vi "Robotics Environment Simulator.vi"() -> ()   [LabVIEW 2013]
doc: "This VI starts and stops the environment simulator and serves as the master VI for your simulation code. Open and run this VI to display the environment simulator, or open the block diagram to view or modify simulation code."
uses:
  <vilib>/Analysis/Matrix/Datatypes/RealMatrix.ctl
  <vilib>/robotics/Simulator/Engine/ctl/Step Mode.ctl
  <vilib>/robotics/Simulator/Engine/ctl/Simulation Mode.ctl
  <vilib>/robotics/Simulator/Engine/ctl/Robot Component ID.ctl
  <resource>/robotics/simulator/Utility/ModelBuilder/Utilities/3DController/Public/ActionType.ctl
  <resource>/robotics/simulator/Utility/ModelBuilder/Utilities/3DController/3DController.lvclass
  SubVIs/SR6-NC Arm/SR6-NC Arm.lvclass
  <instrlib>/Hitec HS400 Series/HAIOL/Hitec HS400 Series.lvclass
  <vilib>/Analysis/baseanly.llb/Real A x B.vi
  <vilib>/Analysis/_algsub.llb/Vector Norm.vi
  <vilib>/Analysis/_algsub.llb/Real Vector Norm.vi
  <vilib>/Analysis/baseanly.llb/Outer Product.vi
  <vilib>/Analysis/baseanly.llb/Real Outer Product.vi
  <vilib>/robotics/Kinematics/Create Lie Group Matrix.vi
  <vilib>/robotics/Simulator/Interface/Simulator References/Get Robot Component Reference.vi
  <vilib>/robotics/Simulator/Interface/Simulator References/Get 3D Visual Scene Reference.vi
  <vilib>/Analysis/baseanly.llb/Real Inverse Matrix.vi
  <vilib>/Analysis/7linalg.llb/Create Special Matrix.vi
  <vilib>/Analysis/7linalg.llb/Create Special Real Matrix.vi
  <vilib>/Analysis/Matrix/Numeric/Multiply/Multiply.vi
  <vilib>/Analysis/Matrix/Numeric/Multiply/Multiply - RM,R.vi
  <vilib>/Analysis/Matrix/Numeric/Multiply/Multiply - R,RM.vi
  <vilib>/Analysis/Matrix/Numeric/Add/Add.vi
  <vilib>/Analysis/Matrix/Numeric/Add/Add - RM,RM.vi
  <vilib>/Analysis/Matrix/Numeric/Subtract/Subtract - RM,RM.vi
  <vilib>/robotics/Kinematics/Robot/Forward Kinematics (Point).vi
  <vilib>/robotics/Simulator/NI_Robotics_Simulator.lvlib
  <instrlib>/Hitec HS400 Series/HAIOL/Simulator/Hitec HS400 Series Simulator.lvclass
  <resource>/objmgr/LVODE.rc
  <vilib>/robotics/Kinematics/NI_Kinematics.lvlib
  <vilib>/Analysis/NI_AALBase.lvlib
  <vilib>/Analysis/Matrix/NI_Matrix.lvlib
panel:
  out "A - B 2":T1
  out "transform":T1
  out "A - B":T1
  out "end effector transform":T1
  out "Ttar":T1
  out "exit":bool
  out "3D Picture":refnum<vi>(3d-picture)
  in  "Joints":dbl[](array[slide])=[0.0, 0.0, 0.0, 0.0, 0.0, -3.673469387755098] scale=-180.0..180.0
  in  "manifest filename":string="Robotics Environment Simulator.xml"
  in  "stop":bool
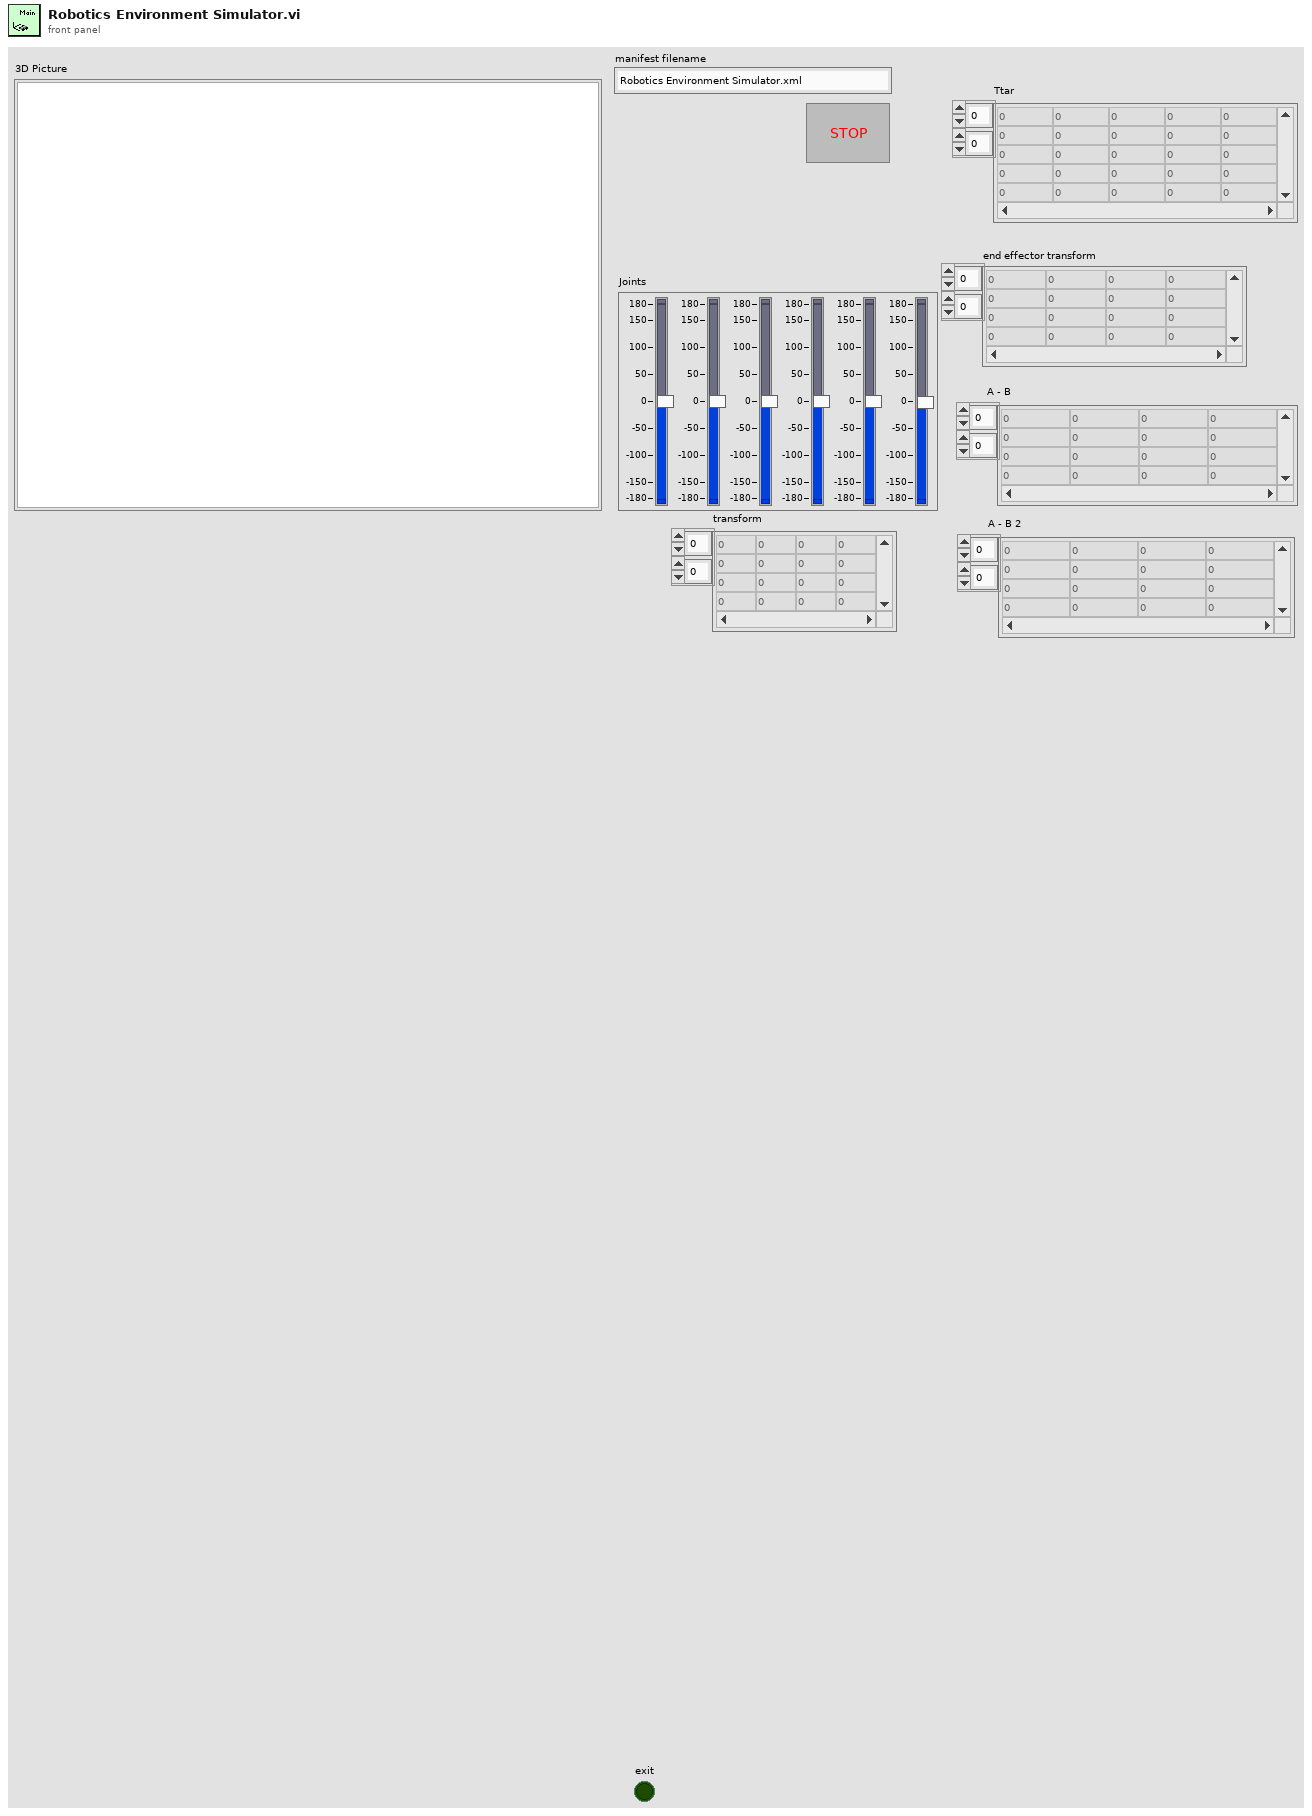
[diagram p1: front panel]
types:
  T1 = typedef "NI_Matrix.lvlib/RealMatrix.ctl" = dbl[][]
  T2 = typedef "NI_Robotics_Simulator.lvlib/Simulation Mode.ctl" = u16
  T3 = typedef "NI_Robotics_Simulator.lvlib/Step Mode.ctl" = u16
  T4 = typedef "NI_Robotics_Simulator.lvlib/Robot Component ID.ctl" = cluster{"robot ID":string, "component ID":string}
  T5 = typedef "NI_Robotics_Model_Builder.lvlib/3DController.lvclass/ActionType.ctl" = enum16{"None", "Trans_X", "Trans_Y", "Trans_Z", "Rot_X", "Rot_Y", "Rot_Z"}
  T6 = cluster{"vector[0]":dbl, "vector[1]":dbl, "vector[2]":dbl}
  T7 = cluster{"Position[0]":sgl, "Position[1]":sgl, "Position[2]":sgl}
  T8 = cluster{"vector":cluster{"vector[0]":dbl, "vector[1]":dbl, "vector[2]":dbl}, "angle":dbl}
  T9 = typedef "LVPoint32TypeDef.ctl" = cluster{"Horizontal":i32, "Vertical":i32}
  T10 = typedef "LV3DPointTypeDef.ctl" = cluster{"X":sgl, "Y":sgl, "Z":sgl}
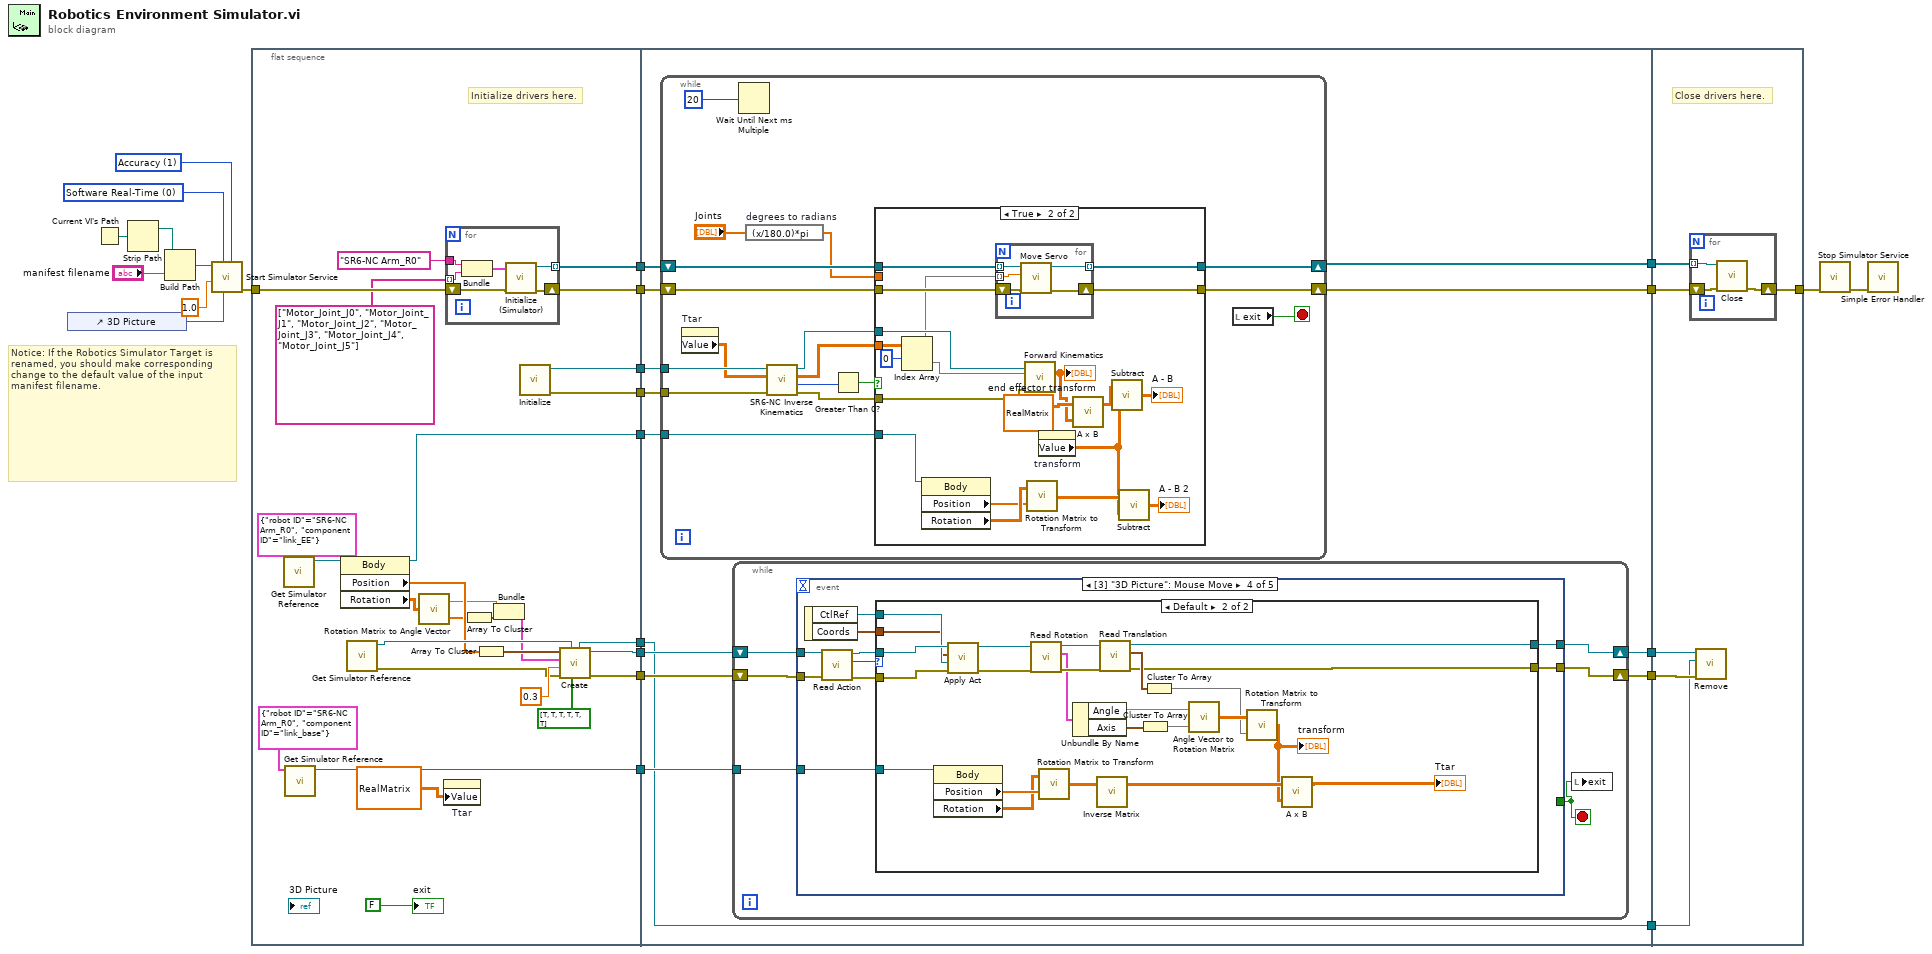
[diagram p0: block diagram]
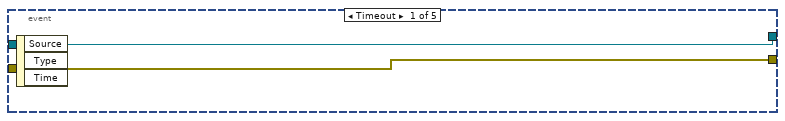
[diagram p2: hidden frame]
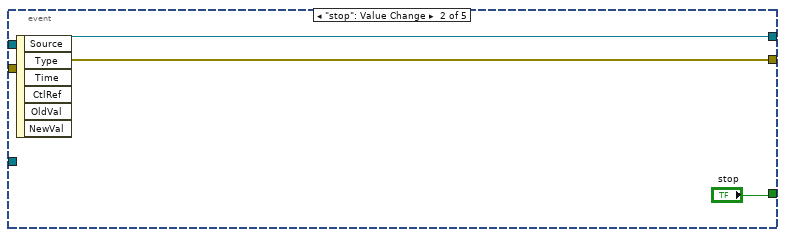
[diagram p3: hidden frame]
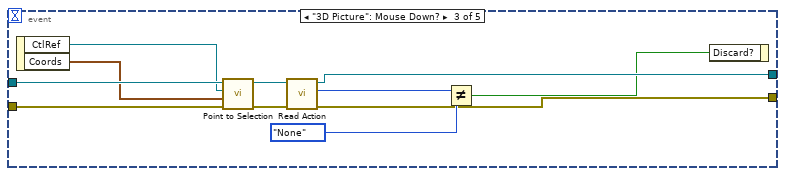
[diagram p4: hidden frame]
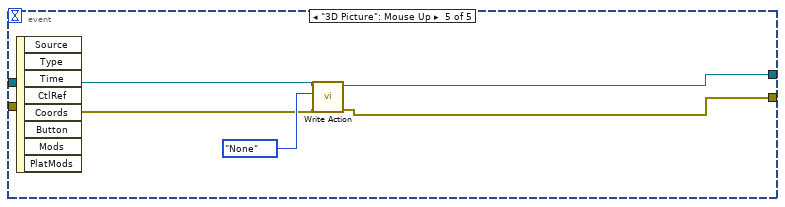
[diagram p6: hidden frame]
diagram:
  w12 = T2 0 items=["Software Real-Time", "Free Running", "Synchronized"] ("timing mode")
  w13 = T3 1 items=["Performance", "Accuracy"] ("step mode")
  # "Notice: If the Robotics Simulator Target is renamed, you should make corresponding change to the default value of the input manifest filename."
  n1 = control-ref of="3D Picture"() -> (w4:refnum<vi>)
  n2 = Current VI's Path() -> (path=w23:path)
  n3 = Strip Path(path=w23) -> (stripped path=w22:path)  [unwired: 1 out]
  n4 = Build Path(base path=w22, name or relative path="manifest filename") -> (appended path=w21:path)
  n5 = call <vilib>:"Start Simulator Service.vi"("step mode"=w13, "3D picture refnum"=w4, "timing mode"=w12, "step size (ms)"=1.0 ("stepsize(ms)"), "manifest file"=w21) -> ("error out"=w18:errorcluster)  [unwired: 6 in]
  n6 = flat-sequence {
    tunnel: w18 -> [w53]
    tunnel: [w52] -> w17
    tunnel: [w49] -> w15
    tunnel: [w35] -> w11
    tunnel: [w34] -> w10
    tunnel: [w33] -> w9
    tunnel: [w31] -> w8
    tunnel: [w29] -> w3
    tunnel: [w28] -> w2
    tunnel: [w26] -> w1
    tunnel: w17 -> [w71]
    tunnel: [w72] -> w16
    tunnel: w15 -> [w70]
    tunnel: [w69] -> w14
    tunnel: w11 -> [w63]
    tunnel: w10 -> [w67]
    tunnel: w9 -> [w68]
    tunnel: w8 -> [w66]
    tunnel: [w65] -> w7
    tunnel: [w64] -> w6
    tunnel: [w63] -> w5
    tunnel: w3 -> [w62]
    tunnel: w2 -> [w61]
    tunnel: w1 -> [w60]
    tunnel: [w182] -> w24
    tunnel: w16 -> [w183]
    tunnel: w14 -> [w184]
    tunnel: w7 -> [w181]
    tunnel: w6 -> [w180]
    tunnel: w5 -> [w179]
    frame #0 {
      # "Initialize drivers here."
      n7 = call-poly <vilib>:"Get Simulator Reference.vi"("robot component ID"=T4 {"robot ID"="SR6-NC Arm_R0", "component ID"="link_EE"}) -> ("component ref"=w42:refnum<k20>)  [unwired: 9 in, 1 out]
      n8 = call-poly <vilib>:"Get Simulator Reference.vi"("robot component ID"=T4 {"robot ID"="SR6-NC Arm_R0", "component ID"="link_base"}) -> ("component ref"=w31:refnum<k20>)  [unwired: 9 in, 1 out]
      n9 = property class="Body"(reference=w42) -> (reference out=w26:refnum<k20>, "Position"=w41:sgl[], "Rotation"=w40:sgl[][])  [unwired: 1 in, 1 out]
      n10 = call-poly <vilib>:"Get Simulator Reference.vi"() -> ("error out"=w43:errorcluster, "scene ref"=w44:refnum<vi>)  [unwired: 10 in]
      n11 = call <vilib>:"Rotation Matrix to Angle Vector.vi"("rotation matrix"=w40) -> ("angle"=w37:dbl, "vector"=w39:dbl[])
      n12 = property on="Ttar" class="Arr (strict)"("Value"=T1 [[1.0, 0.0, 0.0, 0.875], [0.0, 1.0, 0.0, 0.0], [0.0, 0.0, 1.0, 1.215], [0.0, 0.0, 0.0, 0.9999999999999997]] ("Ttar")) -> ()  [unwired: 2 in, 2 out]
      n13 = for {
        shift-right: [w58] -> w52
        shift-left: w53 -> [w59]
        tunnel: "SR6-NC Arm_R0" -> [w57]
        tunnel: string[] ["Motor_Joint_J0", "Motor_Joint_J1", "Motor_Joint_J2", "Motor_Joint_J3", "Motor_Joint_J4", "Motor_Joint_J5"] -> [w56] mode=indexing
        tunnel: [w54] -> w49 mode=indexing
        n14 = Bundle(w57, w56) -> (w55:cluster{string, string})  [unwired: 1 in]
        n15 = call <instrlib>:"Initialize (Simulator).vi"("error in (no error)"=w59, "Device ID"=w55) -> ("error out"=w58:errorcluster, "Hitec HS400 Series out"=w54:refnum<class "Hitec HS400 Series.lvclass">)  [unwired: 8 in]
      }
      n16 = Array To Cluster(array=w39) -> (cluster=w38:T6)
      n17 = Array To Cluster(array=w41) -> (cluster=w46:T7)
      n18 = Bundle("vector"=w38, "angle"=w37) -> (w36:T8)  [unwired: 1 in]
      n19 = call "Initialize.vi"() -> ("error out"=w28:errorcluster, "SR6-NC Arm out"=w29:refnum<class "SR6-NC Arm.lvclass">)  [unwired: 10 in]
      n20 = call <resource>:"Create.vi"("Marks"=bool[] [TRUE, TRUE, TRUE, TRUE, TRUE, TRUE], "Model Root"=w44, "error in (no error)"=w43, "Scale"=0.3, "Rotation"=w36, "Translation"=w46) -> ("error out"=w34:errorcluster, "3DController"=w33:refnum<class "3DController.lvclass">, "Model Root out"=w35:refnum<vi>)  [unwired: 3 in]
      "exit" <- FALSE ("exit")
    }
    frame #1 {
      n21 = while {
        shift-right: [w151] -> w72
        shift-left: w71 -> [w152]
        shift-right: [w149] -> w69
        shift-left: w70 -> [w150]
        tunnel: w62 -> [w144]
        tunnel: w61 -> [w143]
        tunnel: w60 -> [w136]
        stop <- w145 stop-if-true
        n22 = property on="Ttar" class="Arr (strict)"() -> ("Value"=w137:T1)  [unwired: 2 in, 2 out]
        n23 = Wait Until Next ms Multiple(millisecond multiple=20) -> ()  [unwired: 1 out]
        n24 = expression code="(x/180.0)*pi" "degrees to radians"("Joints") -> (w147:dbl[])
        n25 = call-dynamic "SR6-NC Inverse Kinematics.vi"("error in (no error)"=w143, "end effector transform"=w137, "SR6-NC Arm in"=w144) -> ("error out"=w138:errorcluster, "number of valid solutions"=w142:i32, "joint positions"=w140:T1, "SR6-NC Arm out"=w139:refnum<class "SR6-NC Arm.lvclass">)  [unwired: 5 in]
        n26 = Greater Than 0?(x=w142) -> (x > 0?=w141:bool)
        n27 = case shown="True" w141 {
          tunnel: w152 -> [w153 w173]
          tunnel: [w153 w172] -> w151
          tunnel: w150 -> [w154 w171]
          tunnel: [w154 w170] -> w149
          tunnel: w147 -> [_ _]
          tunnel: w140 -> [_ w169]
          tunnel: w139 -> [_ w167]
          tunnel: w138 -> [_ w165]
          tunnel: w136 -> [_ w158]
          frame False {
          }
          frame True {
            n28 = Index Array(array=w169, index (row)=0) -> (element=w166:dbl[])  [unwired: 1 in]
            n29 = property class="Body"(reference=w158) -> ("Position"=w159:sgl[], "Rotation"=w160:sgl[][])  [unwired: 1 in, 2 out]
            n30 = for {
              tunnel: w171 -> [w177] mode=indexing
              shift-right: [w176] -> w172
              shift-left: w173 -> [w178]
              tunnel: [w175] -> w170 mode=indexing
              tunnel: w166 -> [w174] mode=indexing
              n31 = call-dynamic "Move Servo.vi"("error in (no error)"=w178, "CCW Position (0.0 rad)"=w174, "Hitec HS400 Series in"=w177) -> ("error out"=w176:errorcluster, "Hitec HS400 Series out"=w175:refnum<class "Hitec HS400 Series.lvclass">)  [unwired: 7 in]
            }
            n32 = call-poly <vilib>:"Forward Kinematics.vi"("error in (no error)"=w165, "joint positions"=w166, "serial arm in"=w167) -> ("end effector transform"=w162:T1)  [unwired: 6 in, 2 out]
            "end effector transform" <- w162
            n33 = call <vilib>:"Rotation Matrix to Transform.vi"("translation vector"=w159, "rotation matrix"=w160) -> ("transform"=w157:T1)
            n34 = property on="transform" class="Arr (strict)"() -> ("Value"=w156:T1)  [unwired: 2 in, 2 out]
            n35 = call-poly <vilib>:"A x B.vi"("B"=w162, "A"=T1 [[0.9999999403953552, -0.00030462999711744487, 0.0, 1.0], [0.00030462999711744487, 0.9999999403953552, 0.0, 3.0], [0.0, 0.0, 1.0, 0.0], [0.0, 0.0, 0.0, 1.0]] ("Inverse Matrix")) -> ("A x B"=w161:T1)  [unwired: 1 out]
            n36 = call-poly <vilib>:"Subtract.vi"("Real Matrix B"=w156, "Real Matrix A"=w161) -> ("A - B"=→"A - B":T1)
            n37 = call-poly <vilib>:"Subtract.vi"("Real Matrix B"=w156, "Real Matrix A"=w157) -> ("A - B"=→"A - B 2":T1)
          }
        }
        n38 = local read "exit"() -> (w145:bool)
      }
      n39 = while {
        shift-right: [w76] -> w64
        shift-left: w68 -> [w78]
        shift-right: [w75] -> w65
        shift-left: w67 -> [w77]
        tunnel: w66 -> [w74]
        stop <- w73 stop-if-true
        n40 = event shown="[3] \"3D Picture\": Mouse Move" {
          selector: _ -> [_ _ _ _ _]
          dyn-events: _ -> [_ _ _ _ _]
          timeout: _ -> [_ _ _ _ _]
          tunnel: w78 -> [w80 w83 w90 w104 w134]
          tunnel: w77 -> [w79 w82 w89 w103 w133]
          tunnel: [w80 w83 w86 w96 w132] -> w76
          tunnel: [w79 w82 w85 w95 w131] -> w75
          tunnel: w74 -> [_ _ _ w97 _]
          tunnel: [_ "stop" _ _ _] -> w73
          event Timeout {
            n41 = event-data() -> ()  [unwired: 1 in, 3 out]
          }
          event "stop": Value Change {
            n42 = event-data() -> ()  [unwired: 1 in, 6 out]
          }
          event "3D Picture": Mouse Down? {
            n43 = event-data() -> ("CtlRef"=w88:refnum<vi>, "Coords"=w87:T9)  [unwired: 1 in]
            n44 = call-dynamic "Point to Selection.vi"("error in (no error)"=w89, "Coords"=w87, "CtlRef"=w88, "3DController in"=w90) -> ("error out"=w94:errorcluster, "3DController out"=w93:refnum<class "3DController.lvclass">)  [unwired: 6 in]
            n45 = call-dynamic "Read Action.vi"("error in (no error)"=w94, "3DController in"=w93) -> ("error out"=w85:errorcluster, "Action"=w92:T5, "3DController out"=w86:refnum<class "3DController.lvclass">)  [unwired: 7 in]
            n46 = Not Equal?(x=w92, y=ActionType."None") -> (x != y?=w84:bool)
            n47 = event-data("Discard?"=w84) -> ()  [unwired: 1 in, 1 out]
          }
          event "3D Picture": Mouse Move {
            n48 = event-data() -> ("CtlRef"=w99:refnum<vi>, "Coords"=w98:T9)  [unwired: 1 in]
            n49 = call-dynamic "Read Action.vi"("error in (no error)"=w103, "3DController in"=w104) -> ("error out"=w100:errorcluster, "Action"=w102:T5, "3DController out"=w101:refnum<class "3DController.lvclass">)  [unwired: 7 in]
            n50 = case shown="Default" w102 {
              tunnel: w101 -> [w106 w115]
              tunnel: w100 -> [w105 w114]
              tunnel: w99 -> [_ w113]
              tunnel: w98 -> [_ w112]
              tunnel: w97 -> [_ w111]
              tunnel: [w106 w110] -> w96
              tunnel: [w105 w109] -> w95
              frame "None" {
              }
              frame Default {
                n51 = property class="Body"(reference=w111) -> ("Position"=w119:sgl[], "Rotation"=w118:sgl[][])  [unwired: 1 in, 2 out]
                n52 = call-dynamic "Apply Act.vi"("error in (no error)"=w114, "3D Scene"=w113, "End Point"=w112, "3DController in"=w115) -> ("error out"=w129:errorcluster, "3DController out"=w130:refnum<class "3DController.lvclass">)  [unwired: 6 in]
                n53 = call-dynamic "Read Rotation.vi"("error in (no error)"=w129, "3DController in"=w130) -> ("error out"=w127:errorcluster, "Rotation"=w126:cluster{"Axis":T10, "Angle":sgl}, "3DController out"=w128:refnum<class "3DController.lvclass">)  [unwired: 7 in]
                n54 = call <vilib>:"Rotation Matrix to Transform.vi"("translation vector"=w119, "rotation matrix"=w118) -> ("transform"=w107:T1)
                n55 = Unbundle By Name(w126) -> ("Angle"=w123:sgl, "Axis"=w125:T10)
                n56 = call-poly <vilib>:"Inverse Matrix.vi"("Input Matrix"=w107) -> ("Inverse Matrix"=w117:T1)  [unwired: 1 in, 1 out]
                n57 = call-dynamic "Read Translation.vi"("error in (no error)"=w127, "3DController in"=w128) -> ("error out"=w109:errorcluster, "3D Point"=w121:T10, "3DController out"=w110:refnum<class "3DController.lvclass">)  [unwired: 7 in]
                n58 = Cluster To Array(cluster=w125) -> (array=w124:sgl[])
                n59 = Cluster To Array(cluster=w121) -> (array=w120:sgl[])
                n60 = call <vilib>:"Angle Vector to Rotation Matrix.vi"("vector"=w124, "angle"=w123) -> ("rotation matrix"=w122:T1)
                n61 = call <vilib>:"Rotation Matrix to Transform.vi"("translation vector"=w120, "rotation matrix"=w122) -> ("transform"=w116:T1)
                "transform" <- w116
                n62 = call-poly <vilib>:"A x B.vi"("B"=w116, "A"=w117) -> ("A x B"=→"Ttar":T1)  [unwired: 1 out]
              }
            }
          }
          event "3D Picture": Mouse Up {
            n63 = event-data() -> ()  [unwired: 1 in, 8 out]
            n64 = call-dynamic "Write Action.vi"("error in (no error)"=w133, "Action"=ActionType."None", "3DController in"=w134) -> ("error out"=w131:errorcluster, "3DController out"=w132:refnum<class "3DController.lvclass">)  [unwired: 7 in]
          }
        }
        n65 = local write "exit"(w73) -> ()
      }
    }
    frame #2 {
      # "Close drivers here."
      n66 = for {
        tunnel: w184 -> [w187] mode=indexing
        shift-right: [w185] -> w182
        shift-left: w183 -> [w186]
        n67 = call-dynamic "Close.vi"("error in (no error)"=w186, "Hitec HS400 Series in"=w187) -> ("error out"=w185:errorcluster)  [unwired: 9 in]
      }
      n68 = call-dynamic "Remove.vi"("error in (no error)"=w181, "Model Root"=w179, "3DController in"=w180) -> ()  [unwired: 7 in, 2 out]
    }
  }
  n69 = call <vilib>:"Stop Simulator Service.vi"("error in (no error)"=w24) -> ("error out"=w19:errorcluster)  [unwired: 10 in]
  n70 = call <vilib>:"Simple Error Handler.vi"("error in (no error)"=w19) -> ()  [unwired: 4 in, 5 out]
